vi "Read Roles.vi"(8 "error in (no error)":errorcluster, 11 "ACBPassPlay in":refnum<class "ACBPassPlay.lvclass">) -> (0 "error out":errorcluster, 2 "Roles":T1, 3 "ACBPassPlay out":refnum<class "ACBPassPlay.lvclass">)   [LabVIEW 2023, in "ACBPassPlay.lvclass"]
uses:
  ACBPassPlay.lvclass
  ABCSecondKicker_class/ABCSecondKicker.lvclass
  ABCThirdKicker_class/ABCThirdKicker.lvclass
  ABCFirstKickerRole_class/ABCFirstKickerRole.lvclass
  ACBPassPlay.lvclass/ACBPassPlay.ctl
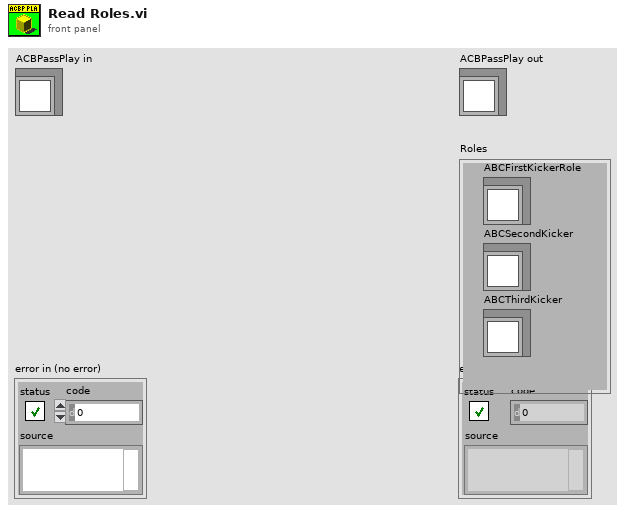
[diagram p1: front panel]
types:
  T1 = cluster{"ABCSecondKicker":refnum<class "ABCSecondKicker.lvclass">, "ABCThirdKicker":refnum<class "ABCThirdKicker.lvclass">, "ABCFirstKickerRole":refnum<class "ABCFirstKickerRole.lvclass">}
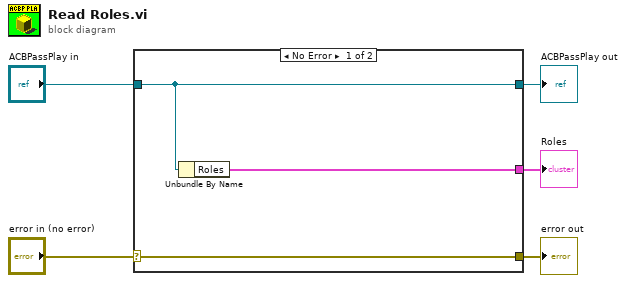
[diagram p0: block diagram]
diagram:
  n1 = case shown="No Error" "error in (no error)" {
    selector: "error in (no error)" -> [w8 w9]
    tunnel: [w8 w9] -> w4
    tunnel: [w7 w10] -> w2
    tunnel: "ACBPassPlay in" -> [w7 w10]
    tunnel: [w6 _] -> w1
    frame No Error {
      n2 = Unbundle By Name(w7) -> ("Roles"=w6:T1)
    }
    frame Error {
    }
  }
  "error out" <- w4
  "ACBPassPlay out" <- w2
  "Roles" <- w1
